vi "GetServiceProviderXML.vi"(9 "Method Name":string="registerService", 11 "ROS":T1) -> (1 "URI":string, 2 "Method Name":string, 3 "lookupService":string)   [LabVIEW 2016]
doc: "Returns the XML for a given service provider"
uses:
  _ROSControl.ctl
  _ROSDirection.ctl
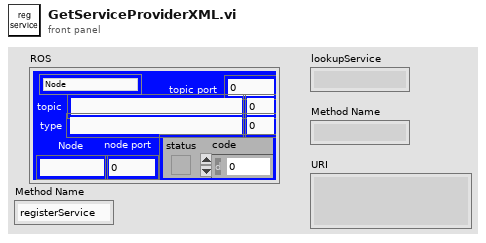
[diagram p1: front panel]
types:
  T1 = typedef "_ROSControl.ctl" = cluster{"topic port":u16, "Node":string, "topic":string, "type":string, "node port":u16, "error ":errorcluster, "Direction":T2, "Update (ms)":u16, "FIFO size":u16}
  T2 = typedef "_ROSDirection.ctl" = enum16{"Node", "Publisher", "Subscriber", "ServiceClient", "ServiceProvider"}
  T3 = enum16{"rosrpc://IP:port", "http://IP:port", "http://IP", "IP:port", "IP only"}
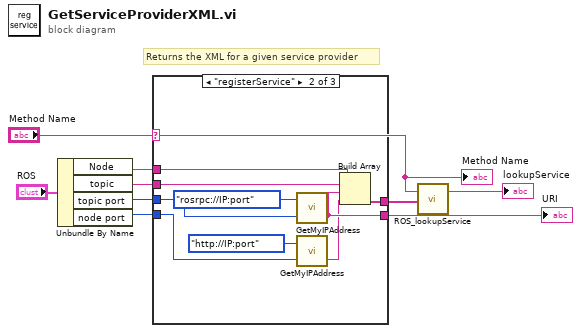
[diagram p0: block diagram]
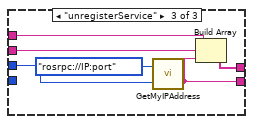
[diagram p3: hidden frame]
diagram:
  # "Returns the XML for a given service provider"
  n1 = Unbundle By Name("ROS") -> ("Node"=w3:string, "topic"=w4:string, "topic port"=w7:u16, "node port"=w5:u16)
  n2 = case shown="\"registerService\"" "Method Name" {
    tunnel: [_ w18 w24] -> w9
    tunnel: [_ w17 w23] -> w8
    tunnel: w7 -> [_ w16 w22]
    tunnel: w5 -> [_ w14 _]
    tunnel: w4 -> [_ w13 w21]
    tunnel: w3 -> [_ w12 w20]
    frame Default {
    }
    frame "registerService" {
      n3 = call "GetMyIPAddress.vi"("Port"=w16, "Format"=T3."rosrpc://IP:port") -> ("URI"=w18:string)  [unwired: 1 out]
      n4 = call "GetMyIPAddress.vi"("Port"=w14, "Format"=T3."http://IP:port") -> ("URI"=w15:string)  [unwired: 1 out]
      n5 = Build Array(w12, w13, w18, w15) -> (w17:string[])
    }
    frame "unregisterService" {
      n6 = call "GetMyIPAddress.vi"("Port"=w22, "Format"=T3."rosrpc://IP:port") -> ("URI"=w24:string)  [unwired: 1 out]
      n7 = Build Array(w20, w21, w24) -> (w23:string[])
    }
  }
  "URI" <- w9
  n8 = call "ROS_lookupService.vi"("Parameters"=w8, "Method Name"="Method Name") -> ("lookupService"=→"lookupService":string)  [unwired: 1 in]
  "Method Name" <- "Method Name"
